vi "SwerveDrivePoseEst2_UpdateWithTime.vi"(6 "CurrentTimeSeconds":dbl=-1.0, 9 "module Positions":T1[](array[typedef]) {"Angle"."SIN" format="%13.4f"; "Angle"."COS" format="%13.4f"; "Angle"."VALUE" format="%13.4f"}, 10 "GyroAngle":T2={"VALUE"=0.0, "COS"=1.0, "SIN"=0.0} {"SIN" format="%13.4f"; "COS" format="%13.4f"; "VALUE" format="%13.4f"}, 11 "in SwerveDrivePoseEst2":T5={"M_Vision_K"=[], "m_nominal_dT"=0.0, "m_PrevTime_Sec"=0.0, "Pose_Buffer"={"TimeStamps"=[], "DataArray"=[], "Min_TimeStamp"=0.0, "Max_TimeStamp"=0.0, "ItemCount"=0, "MaxBufferTime"=0.0}, "Swerve_Drive_Kinematics"={"NumModules"=0, "InverseKinematics"=[], "ForwardKinematics"=[], "Modules"=[], "PrevCoR"={"X"=0.0, "Y"=0.0}, "SavedModuleStates"=[]}, "Swerve_Drive_Odom"={"POSE"={"TRANSLATION"={"X"=0.0, "Y"=0.0}, "ROTATION"={"VALUE"=0.0, "COS"=1.0, "SIN"=0.0}}, "GyroOffset"={"VALUE"=0.0, "COS"=1.0, "SIN"=0.0}, "PreviousAngle"={"VALUE"=0.0, "COS"=1.0, "SIN"=0.0}, "PrevModulePositions"=[], "NumModules"=0}, "M_Q"=[[0.0], [0.0], [0.0]], "NumModules"=-1} {"Swerve_Drive_Odom"."PrevModulePositions"."Angle"."SIN" format="%13.4f"; "Swerve_Drive_Odom"."PrevModulePositions"."Angle"."COS" format="%13.4f"; "Swerve_Drive_Odom"."PrevModulePositions"."Angle"."VALUE" format="%13.4f"; "Swerve_Drive_Odom"."PreviousAngle"."SIN" format="%13.4f"; "Swerve_Drive_Odom"."PreviousAngle"."COS" format="%13.4f"; "Swerve_Drive_Odom"."PreviousAngle"."VALUE" format="%13.4f"; "Swerve_Drive_Odom"."GyroOffset"."SIN" format="%13.4f"; "Swerve_Drive_Odom"."GyroOffset"."COS" format="%13.4f"; "Swerve_Drive_Odom"."GyroOffset"."VALUE" format="%13.4f"; "Swerve_Drive_Odom"."POSE"."ROTATION"."SIN" format="%13.4f"; "Swerve_Drive_Odom"."POSE"."ROTATION"."COS" format="%13.4f"; "Swerve_Drive_Odom"."POSE"."ROTATION"."VALUE" format="%13.4f"; "Swerve_Drive_Odom"."POSE"."TRANSLATION"."Y" format="%14.3f"; "Swerve_Drive_Odom"."POSE"."TRANSLATION"."X" format="%14.3f"; "Swerve_Drive_Kinematics"."SavedModuleStates"."Angle"."SIN" format="%13.4f"; "Swerve_Drive_Kinematics"."SavedModuleStates"."Angle"."COS" format="%13.4f"; "Swerve_Drive_Kinematics"."SavedModuleStates"."Angle"."VALUE" format="%13.4f"; "Swerve_Drive_Kinematics"."PrevCoR"."Y" format="%14.3f"; "Swerve_Drive_Kinematics"."PrevCoR"."X" format="%14.3f"; "Swerve_Drive_Kinematics"."Modules"."Y" format="%14.3f"; "Swerve_Drive_Kinematics"."Modules"."X" format="%14.3f"}) -> (0 "Error":bool, 2 "Estimated Pose":T3 {"ROTATION"."SIN" format="%13.4f"; "ROTATION"."COS" format="%13.4f"; "ROTATION"."VALUE" format="%13.4f"; "TRANSLATION"."Y" format="%14.3f"; "TRANSLATION"."X" format="%14.3f"}, 3 "Out SwerveDrivePoseEst2":T5={"M_Vision_K"=[], "m_nominal_dT"=0.0, "m_PrevTime_Sec"=0.0, "Pose_Buffer"={"TimeStamps"=[], "DataArray"=[], "Min_TimeStamp"=0.0, "Max_TimeStamp"=0.0, "ItemCount"=0, "MaxBufferTime"=0.0}, "Swerve_Drive_Kinematics"={"NumModules"=0, "InverseKinematics"=[], "ForwardKinematics"=[], "Modules"=[], "PrevCoR"={"X"=0.0, "Y"=0.0}, "SavedModuleStates"=[]}, "Swerve_Drive_Odom"={"POSE"={"TRANSLATION"={"X"=0.0, "Y"=0.0}, "ROTATION"={"VALUE"=0.0, "COS"=1.0, "SIN"=0.0}}, "GyroOffset"={"VALUE"=0.0, "COS"=1.0, "SIN"=0.0}, "PreviousAngle"={"VALUE"=0.0, "COS"=1.0, "SIN"=0.0}, "PrevModulePositions"=[], "NumModules"=0}, "M_Q"=[[0.0], [0.0], [0.0]], "NumModules"=-1} {"Swerve_Drive_Odom"."PrevModulePositions"."Angle"."SIN" format="%13.4f"; "Swerve_Drive_Odom"."PrevModulePositions"."Angle"."COS" format="%13.4f"; "Swerve_Drive_Odom"."PrevModulePositions"."Angle"."VALUE" format="%13.4f"; "Swerve_Drive_Odom"."PreviousAngle"."SIN" format="%13.4f"; "Swerve_Drive_Odom"."PreviousAngle"."COS" format="%13.4f"; "Swerve_Drive_Odom"."PreviousAngle"."VALUE" format="%13.4f"; "Swerve_Drive_Odom"."GyroOffset"."SIN" format="%13.4f"; "Swerve_Drive_Odom"."GyroOffset"."COS" format="%13.4f"; "Swerve_Drive_Odom"."GyroOffset"."VALUE" format="%13.4f"; "Swerve_Drive_Odom"."POSE"."ROTATION"."SIN" format="%13.4f"; "Swerve_Drive_Odom"."POSE"."ROTATION"."COS" format="%13.4f"; "Swerve_Drive_Odom"."POSE"."ROTATION"."VALUE" format="%13.4f"; "Swerve_Drive_Odom"."POSE"."TRANSLATION"."Y" format="%14.3f"; "Swerve_Drive_Odom"."POSE"."TRANSLATION"."X" format="%14.3f"; "Swerve_Drive_Kinematics"."SavedModuleStates"."Angle"."SIN" format="%13.4f"; "Swerve_Drive_Kinematics"."SavedModuleStates"."Angle"."COS" format="%13.4f"; "Swerve_Drive_Kinematics"."SavedModuleStates"."Angle"."VALUE" format="%13.4f"; "Swerve_Drive_Kinematics"."PrevCoR"."Y" format="%14.3f"; "Swerve_Drive_Kinematics"."PrevCoR"."X" format="%14.3f"; "Swerve_Drive_Kinematics"."Modules"."Y" format="%14.3f"; "Swerve_Drive_Kinematics"."Modules"."X" format="%14.3f"})   [LabVIEW 2019, in "Trajectory_Library.lvlib"]
doc: "Updates the the robot odometry using only wheel encoder information. Note that this should be called every loop.\n\nInputs:\n - inSwerveDrivePoseEst -- system data cluster\n - gyroAngle -- The current gyro angle. (radians)\n - ModulePositions -- Array Module Position -- The current module positions (distance and angle)\n - currentTime -- Time at which this method was called, in seconds.\n\nOutputs:\n - outSwerveDrivePoseEst -- system data cluster\n - EstimatedPose -- The estimated pose of the robot in meters."
uses:
  Trajectory_Library.lvlib
  <vilib>/Analysis/Matrix/Datatypes/RealMatrix.ctl
  <vilib>/Analysis/Matrix/NI_Matrix.lvlib
  TypeDef/ROTATION2D.ctl
  TypeDef/TRANSLATION2D.ctl
  TypeDef/POSE2D.ctl
  TypeDef/TIME_INTERPOLATABLE_VARIANT.ctl
  TypeDef/SWERVE_DRIVE_MODULE_STATE.ctl
  TypeDef/SWERVE_DRIVE_KINEMATICS.ctl
  TypeDef/SWERVE_DRIVE_MODULE_POSITION.ctl
  TypeDef/SWERVE_DRIVE_ODOMETRY.ctl
  TypeDef/SWERVE_DRIVE_POSE_EST2.ctl
panel:
  # "<3, 1>"
  # "<3, 3>"
  # "<3, 1>"
  # "<3, 3>"
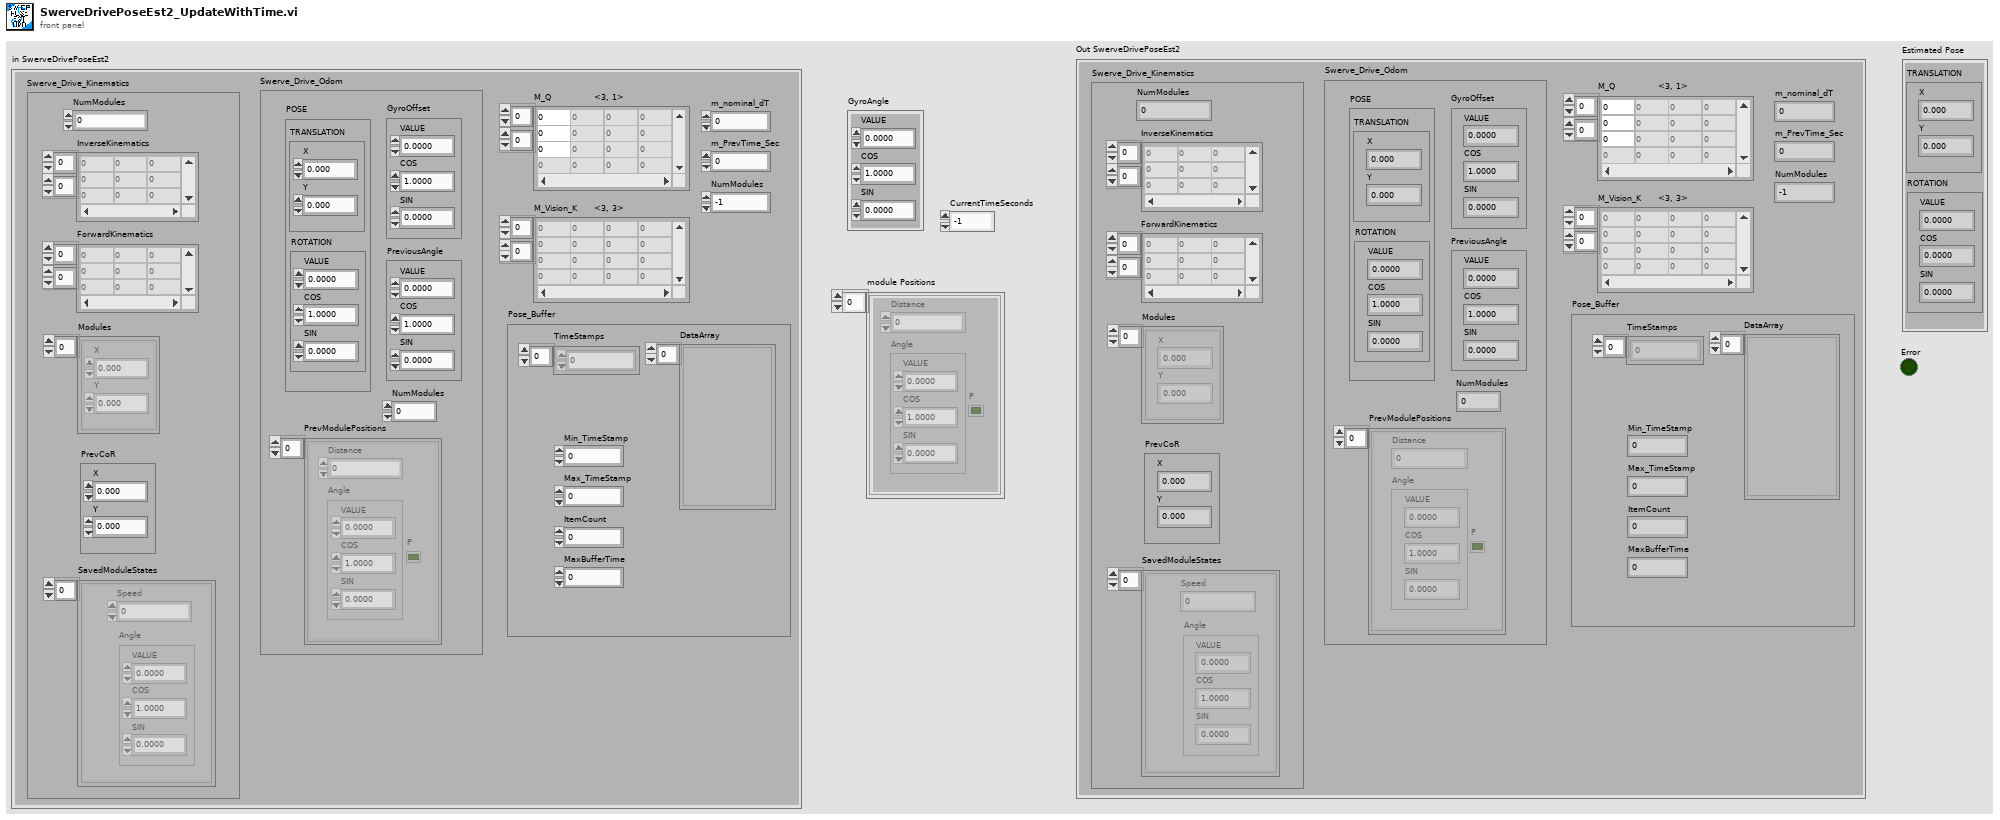
[diagram p1: front panel]
types:
  T1 = typedef "Trajectory_Library.lvlib/SWERVE_DRIVE_MODULE_POSITION.ctl" = cluster{"Distance":dbl, "Angle":T2, "P":bool}
  T2 = typedef "Trajectory_Library.lvlib/ROTATION2D.ctl" = cluster{"VALUE":dbl, "COS":dbl, "SIN":dbl}
  T3 = typedef "Trajectory_Library.lvlib/POSE2D.ctl" = cluster{"TRANSLATION":T4, "ROTATION":T2}
  T4 = typedef "Trajectory_Library.lvlib/TRANSLATION2D.ctl" = cluster{"X":dbl, "Y":dbl}
  T5 = typedef "Trajectory_Library.lvlib/SWERVE_DRIVE_POSE_EST2.ctl" = cluster{"M_Vision_K":T6, "m_nominal_dT":dbl, "m_PrevTime_Sec":dbl, "Pose_Buffer":T7, "Swerve_Drive_Kinematics":T8, "Swerve_Drive_Odom":T10, "M_Q":T6, "NumModules":i32}
  T6 = typedef "NI_Matrix.lvlib/RealMatrix.ctl" = dbl[][]
  T7 = typedef "Trajectory_Library.lvlib/TIME_INTERPOLATABLE_VARIANT.ctl" = cluster{"TimeStamps":dbl[], "DataArray":variant[], "Min_TimeStamp":dbl, "Max_TimeStamp":dbl, "ItemCount":i32, "MaxBufferTime":dbl}
  T8 = typedef "Trajectory_Library.lvlib/SWERVE_DRIVE_KINEMATICS.ctl" = cluster{"NumModules":i32, "InverseKinematics":T6, "ForwardKinematics":T6, "Modules":T4[], "PrevCoR":T4, "SavedModuleStates":T9[]}
  T9 = typedef "Trajectory_Library.lvlib/SWERVE_DRIVE_MODULE_STATE.ctl" = cluster{"Speed":dbl, "Angle":T2}
  T10 = typedef "Trajectory_Library.lvlib/SWERVE_DRIVE_ODOMETRY.ctl" = cluster{"POSE":T3, "GyroOffset":T2, "PreviousAngle":T2, "PrevModulePositions":T1[], "NumModules":i32}
  T11 = typedef "Trajectory_Library.lvlib/SWERVE_DRIVE_POSE_EST2_INTERP_RECORD.ctl" = cluster{"PoseMeters":T3, "GyroAngle":T2, "ModulePositions":T1[]}
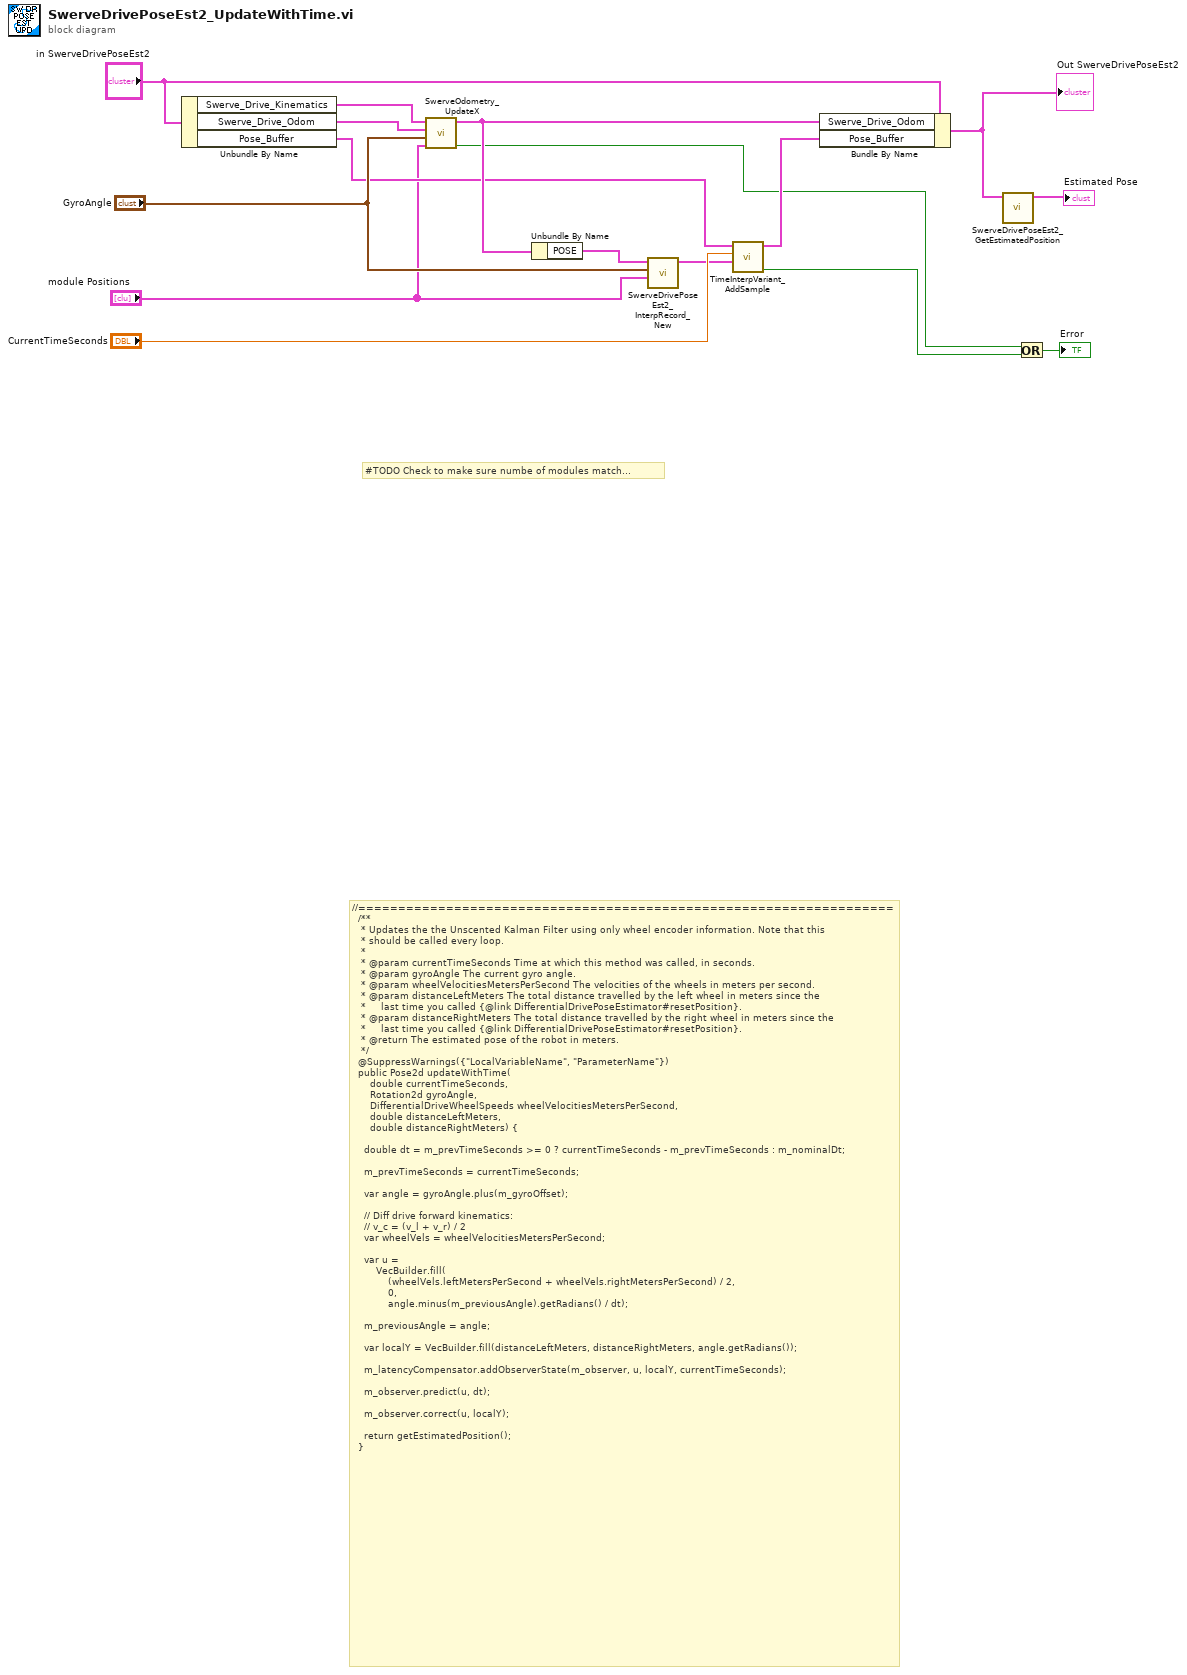
[diagram p0: block diagram]
diagram:
  # "#TODO Check to make sure numbe of modules match..."
  # "//===================================================================\n  /**\n   * Updates the the Unscented Kalman Filter using only wheel encoder information. Note that this\n   * should be called every loop.\n   *\n   * @param currentTimeSeconds Time at which this method was called, in seconds.\n   * @param gyroAngle The current gyro angle.\n   * @param wheelVelocitiesMetersPerSecond The velocities of the wheels in meters per second.\n   * @param distanceLeftMeters The total distance travelled by the left wheel in meters since the\n   *     last time you called {@link DifferentialDrivePoseEstimator#resetPosition}.\n   * @param distanceRightMeters The total distance travelled by the right wheel in meters since the\n   *     last time you called {@link DifferentialDrivePoseEstimator#resetPosition}.\n   * @return The estimated pose of the robot in meters.\n   */\n  @SuppressWarnings({\"LocalVariableName\", \"ParameterName\"})\n  public Pose2d updateWithTime(\n      double currentTimeSeconds,\n      Rotation2d gyroAngle,\n      DifferentialDriveWheelSpeeds wheelVelocitiesMetersPerSecond,\n      double distanceLeftMeters,\n      double distanceRightMeters) {\n\n    double dt = m_prevTimeSeconds >= 0 ? currentTimeSeconds - m_prevTimeSeconds : m_nominalDt;\n\n    m_prevTimeSeconds = currentTimeSeconds;\n\n    var angle = gyroAngle.plus(m_gyroOffset);\n\n    // Diff drive forward kinematics:\n    // v_c = (v_l + v_r) / 2\n    var wheelVels = wheelVelocitiesMetersPerSecond;\n\n    var u =\n        VecBuilder.fill(\n            (wheelVels.leftMetersPerSecond + wheelVels.rightMetersPerSecond) / 2,\n            0,\n            angle.minus(m_previousAngle).getRadians() / dt);\n\n    m_previousAngle = angle;\n\n    var localY = VecBuilder.fill(distanceLeftMeters, distanceRightMeters, angle.getRadians());\n\n    m_latencyCompensator.addObserverState(m_observer, u, localY, currentTimeSeconds);\n\n    m_observer.predict(u, dt);\n\n    m_observer.correct(u, localY);\n\n    return getEstimatedPosition();\n  }"
  n1 = Unbundle By Name("in SwerveDrivePoseEst2") -> ("Swerve_Drive_Kinematics"=w6:T8, "Swerve_Drive_Odom"=w5:T10, "Pose_Buffer"=w12:T7)
  n2 = call "SwerveOdometry_UpdateX.vi"("module Positions"="module Positions", "gyroAngle"="GyroAngle", "in SWERVE_DRIVE_ODOMETRY"=w5, "SWERVE_DRIVE_KINEMATICS"=w6) -> ("Error"=w1:bool, "out SWERVE_DRIVE_ODOMETRY"=w15:T10)  [unwired: 5 in, 1 out]
  n3 = Unbundle By Name(w15) -> ("POSE"=w14:T3)
  n4 = call "SwerveDrivePoseEst2_InterpRecord_New.vi"("ModulePositions"="module Positions", "GyroAngle"="GyroAngle", "M_POSE_Meters"=w14) -> ("SWERVE_DRIVE_POSE_EST2_INTERP_RECORD"=w10:T11)  [unwired: 8 in]
  n5 = call "TimeInterpVariant_AddSample.vi"("Variant"=w10, "TimeStamp"="CurrentTimeSeconds", "in TimeInterpVariant"=w12) -> ("Error"=w2:bool, "out TimeInterpVariant"=w9:T7)  [unwired: 7 in]
  n6 = Bundle By Name(cluster="in SwerveDrivePoseEst2", "Swerve_Drive_Odom"=w15, "Pose_Buffer"=w9) -> (w8:T5)
  "Out SwerveDrivePoseEst2" <- w8
  n7 = call "SwerveDrivePoseEst2_GetEstimatedPosition.vi"("in SwerveDrivePoseEstimate"=w8) -> ("Estimated Pose"=→"Estimated Pose":T3)  [unwired: 10 in]
  n8 = Or(x=w1, y=w2) -> (x .or. y?=→"Error":bool)
